vi "CB Augment Model Input Error.vi"(11 "State Space Model":T1) -> (3 "State Space Model Augmented":T1)   [LabVIEW 2020]
uses:
  CB State Space.ctl
  <vilib>/Analysis/Matrix/Datatypes/RealMatrix.ctl
  <vilib>/Analysis/Matrix/NI_Matrix.lvlib
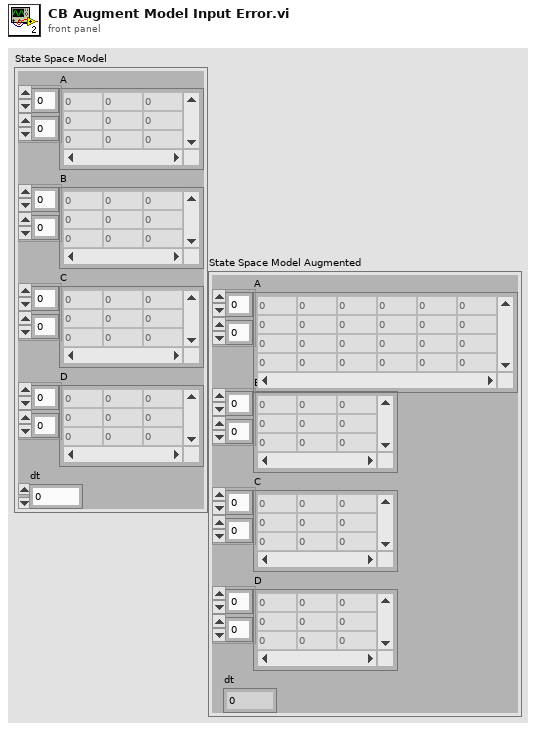
[diagram p1: front panel]
types:
  T1 = typedef "CB State Space.ctl" = cluster{"A":T2, "B":T2, "C":T2, "D":T2, "dt":dbl}
  T2 = typedef "NI_Matrix.lvlib/RealMatrix.ctl" = dbl[][]
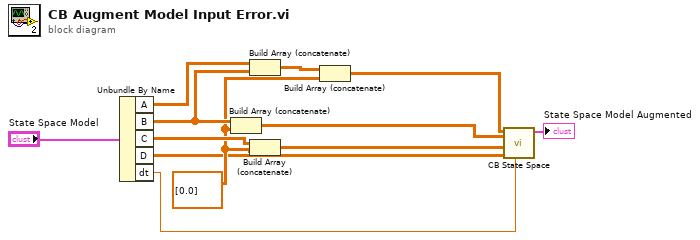
[diagram p0: block diagram]
diagram:
  w7 = T2 [[0.0]] ("array")
  n1 = Unbundle By Name("State Space Model") -> ("A"=w10:T2, "B"=w9:T2, "C"=w11:T2, "D"=w3:T2, "dt"=w2:dbl)
  n2 = Build Array (concatenate)(w9, w7) -> (w5:T2)
  n3 = Build Array (concatenate)(w10, w9) -> (w8:T2)
  n4 = Build Array (concatenate)(w11, w7) -> (w4:T2)
  n5 = Build Array (concatenate)(w8, w7) -> (w6:T2)
  n6 = call "CB State Space.vi"("dt"=w2, "D"=w3, "C"=w4, "B"=w5, "A"=w6) -> ("State Space Model"=→"State Space Model Augmented":T1)  [unwired: 5 in, 1 out]
